vi "Begin.vi"(11 "Image Size":T1=enum."160x120") -> (0 "error out":errorcluster)   [LabVIEW 2013]
doc: "Called before other user functions, this VI is expected to open initial I/O refnums, load in file data, and do all program initialization. Notice that the <B>error out</B> terminal is simply used for data flow. Wiring it to other structures or subVIs ensures that this VI runs first."
uses:
  <vilib>/Rock Robotics/WPI/Camera/WPI_CameraImageSize.ctl
  <vilib>/Rock Robotics/SystemInterfaces/DIO/FPGA_DIOPWMChannel.ctl
  <vilib>/Rock Robotics/WPI/Camera/WPI_CameraWhite Balance Values.ctl
  <vilib>/Rock Robotics/WPI/Camera/WPI_CameraExposure Values.ctl
  <vilib>/Rock Robotics/WPI/Camera/WPI_CameraFrameRate.ctl
  <vilib>/Rock Robotics/WPI/DriverStation/WPI_DriverStationRobotMode2.ctl
  <vilib>/Rock Robotics/WPI/Joystick/WPI_JoystickDeviceEnum.ctl
  <vilib>/Rock Robotics/SystemInterfaces/DIO/FPGA_DIORelayChannel.ctl
  <vilib>/Rock Robotics/WPI/Relay/WPI_RelayDirection.ctl
  <vilib>/Rock Robotics/WPI/SafetyOutput/WPI_SafetyOutputConfigMenu.ctl
  Robot Global Data.vi
  <vilib>/Rock Robotics/WPI/RobotDrive/WPI_RobotDriveOpen2MotorWithVictor.vi
  <vilib>/Rock Robotics/WPI/MotorControl/WPI_MotorControlOpen Talon.vi
  <vilib>/Rock Robotics/WPI/MotorControl/WPI_MotorControlOpen Jaguar.vi
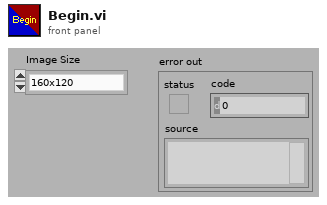
[diagram p1: front panel]
types:
  T1 = typedef "WPI_CameraImageSize.ctl" = enum16{"640x480", "320x240", "160x120"}
  T2 = typedef "WPI_SafetyOutputConfigMenu.ctl" = enum16{"Enable", "Disable"}
  T3 = typedef "WPI_RelayDirection.ctl" = enum16{"Both directions", "Forward only", "Reverse only"}
  T4 = typedef "FPGA_DIORelayChannel.ctl" = enum8{"Relay 1", "Relay 2", "Relay 3", "Relay 4", "Relay 5", "Relay 6", "Relay 7", "Relay 8", "Invalid"}
  T5 = typedef "FPGA_DIOPWMChannel.ctl" = enum8{"PWM 1", "PWM 2", "PWM 3", "PWM 4", "PWM 5", "PWM 6", "PWM 7", "PWM 8", "PWM 9", "PWM 10", "Invalid"}
  T6 = typedef "WPI_JoystickDeviceEnum.ctl" = enum16{"USB 1", "USB 2", "USB 3", "USB 4", "Kinect 1", "Kinect 2"}
  T7 = typedef "WPI_DriverStationRobotMode2.ctl" = enum16{"Autonomous Disabled", "Autonomous Enabled", "Teleop Disabled", "Teleop Enabled", "Timeout", "Finish", "Test Disabled", "Test Enabled"}
  T8 = typedef "WPI_CameraFrameRate.ctl" = u32
  T9 = typedef "WPI_CameraExposure Values.ctl" = enum16{"Auto", "Flicker-free 50 Hz", "Flicker-free 60 Hz", "Hold current"}
  T10 = typedef "WPI_CameraWhite Balance Values.ctl" = enum16{"Auto", "Fixed indoor", "Fixed outdoor 1", "Fixed outdoor 2", "Fixed fluorescent 1", "Fixed fluorescent 2", "Hold current"}
  T11 = typedef "WPI_JoystickDevRef.ctl" = cluster{"Device":T6}
  T12 = typedef "WPI_RobotDriveDevRef.ctl" = cluster{"DevStatus":errorcluster, "Motors[]":T13[], "Square Inputs":bool, "Max Output":dbl, "Isochronous":bool}
  T13 = typedef "WPI_MotorControlDeviceRef.ctl" = cluster{"DeviceStatus":errorcluster, "Type":enum16{"PWM", "CAN"}, "PWM":cluster{"Digital Module":T14, "PWM Channel":T5, "DeadBand":T15}, "CAN":cluster{"Device Number":u8, "Control Mode":T16, "Semaphore":T17, "Max Vout":dbl}, "Invert":bool, "TransformRef":T18, "InvTransformRef":T18}
  T14 = typedef "FPGA_TypedefDigitalModule.ctl" = enum16{"Digital Module 1", "Digital Module 2"}
  T15 = typedef "WPI_PWMDeadband.ctl" = cluster{"Name":string, "maxPositivePwm":i32, "minPositivePwm":i32, "centerPwm":i32, "maxNegativePwm":i32, "minNegativePwm":i32, "angularRange":u16}
  T16 = typedef "WPI_CANJaguar_ControlMode.ctl" = enum8{"Percent VBus", "Current", "Speed", "Position", "Voltage"}
  T17 = typedef "Semaphore RefNum" = refnum<k1>
  T18 = typedef "WPI_PWMTransform_ConPane.ctl" = refnum<vi>
  T19 = typedef "WPI_RelayDevRef.ctl" = cluster{"DevStatus":errorcluster, "Relay Channel":T4, "Digital Module":T14, "Relay Direction":T3}
  T20 = typedef "WPI_CameraDevRef.ctl" = cluster{"Camera Address":string, "CameraStatus":errorcluster, "Acquire Image Notifier":refnum<notifier>}
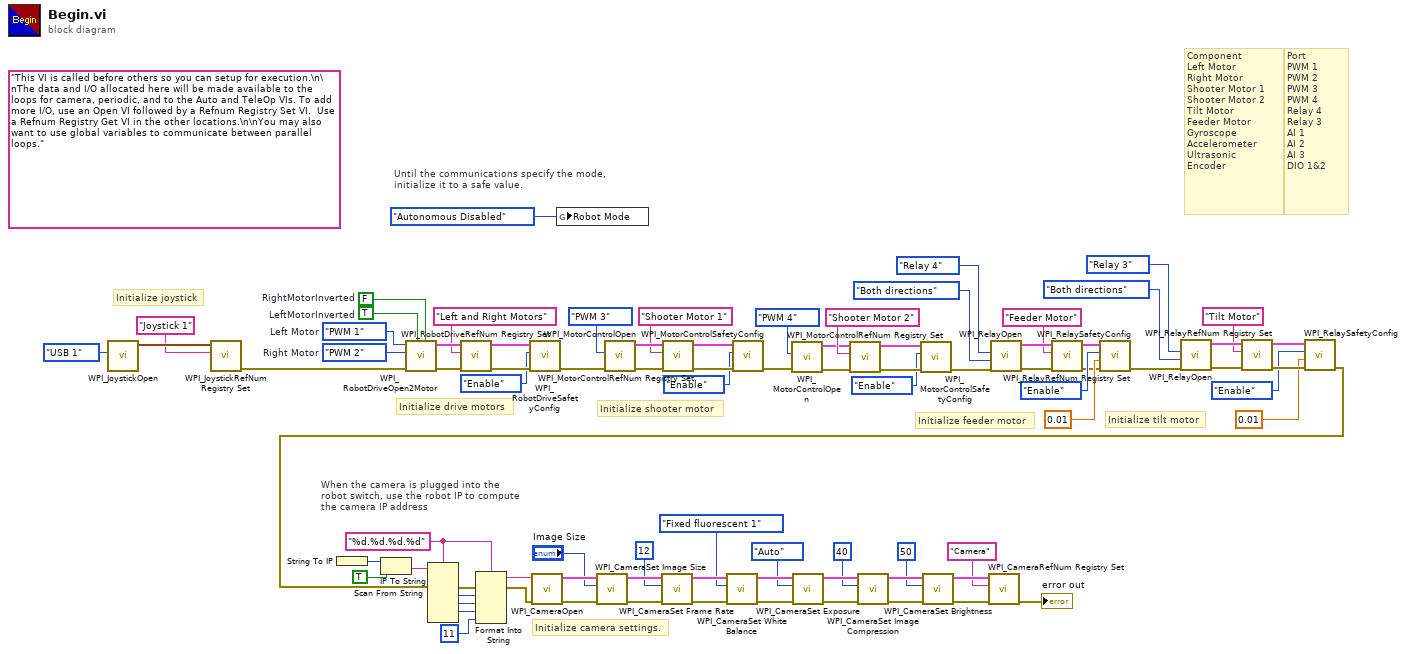
[diagram p0: block diagram]
diagram:
  w54 = "%d.%d.%d.%d" ("format string")
  (unwired) "This VI is called before others so you can setup for execution.\n\nThe data and I/O allocated here will be made available to the loops for camera, periodic, and to the Auto and TeleOp VIs. To add more I/O, use an Open VI followed by a Refnum Registry Set VI.  Use a Refnum Registry Get VI in the other locations.\n\nYou may also want to use global variables to communicate between parallel loops."
  w65 = FPGA_DIOPWMChannel."PWM 2"  # Right Motor
  w34 = FPGA_DIOPWMChannel."PWM 1"  # Left Motor
  w84 = TRUE  # LeftMotorInverted
  w85 = FALSE  # RightMotorInverted
  # "Initialize tilt motor"
  # "Port\nPWM 1\nPWM 2\nPWM 3\nPWM 4\nRelay 4\nRelay 3\nAI 1\nAI 2\nAI 3\nDIO 1&2"
  # "Component\nLeft Motor\nRight Motor\nShooter Motor 1\nShooter Motor 2\nTilt Motor\nFeeder Motor\nGyroscope\nAccelerometer\nUltrasonic\nEncoder"
  # "Initialize feeder motor"
  # "Initialize shooter motor"
  # "Initialize joystick"
  # "Until the communications specify the mode,\ninitialize it to a safe value."
  # "When the camera is plugged into the\nrobot switch, use the robot IP to compute\nthe camera IP address"
  # "Initialize drive motors"
  # "Initialize camera settings."
  n1 = call <vilib>:"WPI_JoystickOpen.vi"("JoystickDevice"=WPI_JoystickDeviceEnum."USB 1") -> ("JoystickDevRef"=w50:T11)  [unwired: 10 out]
  n2 = call <vilib>:"WPI_JoystickRefNum Registry Set.vi"("refnum name"="Joystick 1", "JoystickDevRef"=w50) -> ("error out"=w24:errorcluster)  [unwired: 1 in, 8 out]
  n3 = String To IP() -> (0:w61:u32)  [unwired: 1 in]
  n4 = IP To String(1:TRUE ("dot notation? (F)"), 2:w61) -> (0:w59:string)
  n5 = call-poly <vilib>:"WPI_RobotDriveOpen2Motor.vi"("Right Motor Inverted"=w85, "Left Motor Inverted"=w84, "error in (no error)"=w24, "Right Motor"=w65, "Left Motor"=w34) -> ("error out"=w81:errorcluster, "RobotDriveDevRef"=w83:T12)  [unwired: 5 out]
  n6 = call <vilib>:"WPI_RobotDriveRefNum Registry Set.vi"("error in (no error)"=w81, "refnum name"="Left and Right Motors", "RobotDriveDevRef"=w83) -> ("error out"=w39:errorcluster, "RobotDriveDevRef"=w53:T12)  [unwired: 7 out]
  n7 = call <vilib>:"WPI_RobotDriveSafetyConfig.vi"("error in (no error)"=w39, "mode"=WPI_SafetyOutputConfigMenu."Enable", "RobotDriveDevRef"=w53) -> ("error out"=w33:errorcluster)  [unwired: 7 in, 1 out]
  n8 = global write "Robot Global Data.vi" "Robot Mode"(WPI_DriverStationRobotMode2."Autonomous Disabled" ("Robot Mode")) -> ()
  n9 = call-poly <vilib>:"WPI_MotorControlOpen.vi"("error in (no error)"=w33, "PWM Channel"=FPGA_DIOPWMChannel."PWM 3") -> ("error out"=w38:errorcluster, "MotorControlDeviceRef"=w32:T13)  [unwired: 8 in]
  n10 = call <vilib>:"WPI_MotorControlRefNum Registry Set.vi"("error in (no error)"=w38, "refnum name"="Shooter Motor 1", "MotorControlDevRef"=w32) -> ("error out"=w37:errorcluster, "MotorControlDevRef"=w46:T13)  [unwired: 7 in]
  n11 = call <vilib>:"WPI_MotorControlSafetyConfig.vi"("error in (no error)"=w37, "mode"=WPI_SafetyOutputConfigMenu."Enable", "MotorControlDevRef"=w46) -> ("error out"=w19:errorcluster)  [unwired: 7 in, 1 out]
  n12 = call-poly <vilib>:"WPI_MotorControlOpen.vi"("error in (no error)"=w19, "PWM Channel"=FPGA_DIOPWMChannel."PWM 4") -> ("error out"=w18:errorcluster, "MotorControlDeviceRef"=w21:T13)  [unwired: 8 in]
  n13 = call <vilib>:"WPI_MotorControlRefNum Registry Set.vi"("error in (no error)"=w18, "refnum name"="Shooter Motor 2", "MotorControlDevRef"=w21) -> ("error out"=w15:errorcluster, "MotorControlDevRef"=w12:T13)  [unwired: 7 in]
  n14 = call <vilib>:"WPI_MotorControlSafetyConfig.vi"("error in (no error)"=w15, "mode"=WPI_SafetyOutputConfigMenu."Enable", "MotorControlDevRef"=w12) -> ("error out"=w14:errorcluster)  [unwired: 7 in, 1 out]
  n15 = call <vilib>:"WPI_RelayOpen.vi"("error in (no error)"=w14, "Relay Direction"=WPI_RelayDirection."Both directions", "Relay Channel"=FPGA_DIORelayChannel."Relay 4") -> ("error out"=w36:errorcluster, "RelayDevRef"=w43:T19)  [unwired: 7 in]
  n16 = call <vilib>:"WPI_RelayRefNum Registry Set.vi"("error in (no error)"=w36, "refnum name"="Feeder Motor", "RelayDevRef"=w43) -> ("error out"=w35:errorcluster, "RelayDevRef"=w44:T19)  [unwired: 7 in]
  n17 = call <vilib>:"WPI_RelaySafetyConfig.vi"("error in (no error)"=w35, "timeout (s)"=0.01, "mode"=WPI_SafetyOutputConfigMenu."Enable", "RelayDevRef"=w44) -> ("error out"=w6:errorcluster)  [unwired: 6 in, 1 out]
  n18 = call <vilib>:"WPI_RelayOpen.vi"("error in (no error)"=w6, "Relay Direction"=WPI_RelayDirection."Both directions", "Relay Channel"=FPGA_DIORelayChannel."Relay 3") -> ("error out"=w11:errorcluster, "RelayDevRef"=w10:T19)  [unwired: 7 in]
  n19 = call <vilib>:"WPI_RelayRefNum Registry Set.vi"("error in (no error)"=w11, "refnum name"="Tilt Motor", "RelayDevRef"=w10) -> ("error out"=w5:errorcluster, "RelayDevRef"=w4:T19)  [unwired: 7 in]
  n20 = call <vilib>:"WPI_RelaySafetyConfig.vi"("error in (no error)"=w5, "timeout (s)"=0.01, "mode"=WPI_SafetyOutputConfigMenu."Enable", "RelayDevRef"=w4) -> ("error out"=w1:errorcluster)  [unwired: 6 in, 1 out]
  n21 = Scan From String(format string=w54, input string=w59, error in=w1) -> (error out=w17:errorcluster, output 1=w58:i32, output 2=w57:i32, output 3=w56:i32)  [unwired: 6 in, 2 out]
  n22 = Format Into String(format string=w54, error in=w17, w58, w57, w56, 11 ("Compression")) -> (resulting string=w51:string, error out=w16:errorcluster)  [unwired: 1 in]
  n23 = call <vilib>:"WPI_CameraOpen.vi"("error in (no error)"=w16, "Camera Address"=w51) -> ("error out"=w74:errorcluster, "CameraDevRef"=w75:T20)  [unwired: 8 out]
  n24 = call <vilib>:"WPI_CameraSet Image Size.vi"("error in (no error)"=w74, "Image Size"="Image Size", "CameraDevRef"=w75) -> ("error out"=w73:errorcluster, "CameraDevRef Out"=w76:T20)  [unwired: 7 out]
  n25 = call <vilib>:"WPI_CameraSet Frame Rate.vi"("error in (no error)"=w73, "Frame Rate (fps)"=T8 12, "CameraDevRef"=w76) -> ("error out"=w72:errorcluster, "CameraDevRef Out"=w78:T20)  [unwired: 7 out]
  n26 = call <vilib>:"WPI_CameraSet White Balance.vi"("error in (no error)"=w72, "White Balance"=WPI_CameraWhite_Balance_Values."Fixed fluorescent 1", "CameraDevRef"=w78) -> ("error out"=w71:errorcluster, "CameraDevRef Out"=w77:T20)  [unwired: 7 out]
  n27 = call <vilib>:"WPI_CameraSet Exposure.vi"("error in (no error)"=w71, "Exposure"=WPI_CameraExposure_Values."Auto", "CameraDevRef"=w77) -> ("error out"=w70:errorcluster, "CameraDevRef Out"=w80:T20)  [unwired: 7 out]
  n28 = call <vilib>:"WPI_CameraSet Image Compression.vi"("error in (no error)"=w70, "Compression"=40, "CameraDevRef"=w80) -> ("error out"=w69:errorcluster, "CameraDevRef Out"=w79:T20)  [unwired: 7 out]
  n29 = call <vilib>:"WPI_CameraSet Brightness.vi"("error in (no error)"=w69, "Brightness"=50, "CameraDevRef"=w79) -> ("error out"=w67:errorcluster, "CameraDevRef Out"=w68:T20)  [unwired: 7 out]
  n30 = call <vilib>:"WPI_CameraRefNum Registry Set.vi"("error in (no error)"=w67, "refnum name"="Camera", "CameraDevRef"=w68) -> ("error out"=→"error out":errorcluster)  [unwired: 8 out]
